vi "Voorbeeld_max_2_freq_detection.vi"() -> ()   [LabVIEW 2019]
uses:
  <vilib>/express/express analysis/Spectral/Block/exnSpectralBlock spectral measurements power poly.vi
  <vilib>/express/express analysis/Spectral/Block/exnSpectralBlock spectral measurements power DDT.vi
  <vilib>/express/express analysis/Spectral/XNode/ExpressSpectralMeasurementsBlockNode.xnode
panel:
  in  "Test Freq 2":dbl=1000.0 caption="Frequency"
  in  "Test Freq 1":dbl=500.0 caption="Frequency"
  in  "stop":bool
  out "Freq 2":i32
  out "Freq 1":i32
  out "Fourier Size":i32
  out "Waveform Graph 2":dynamicdata(graph)
  out "Frequency":dbl
  out "Waveform Graph":dynamicdata(graph)
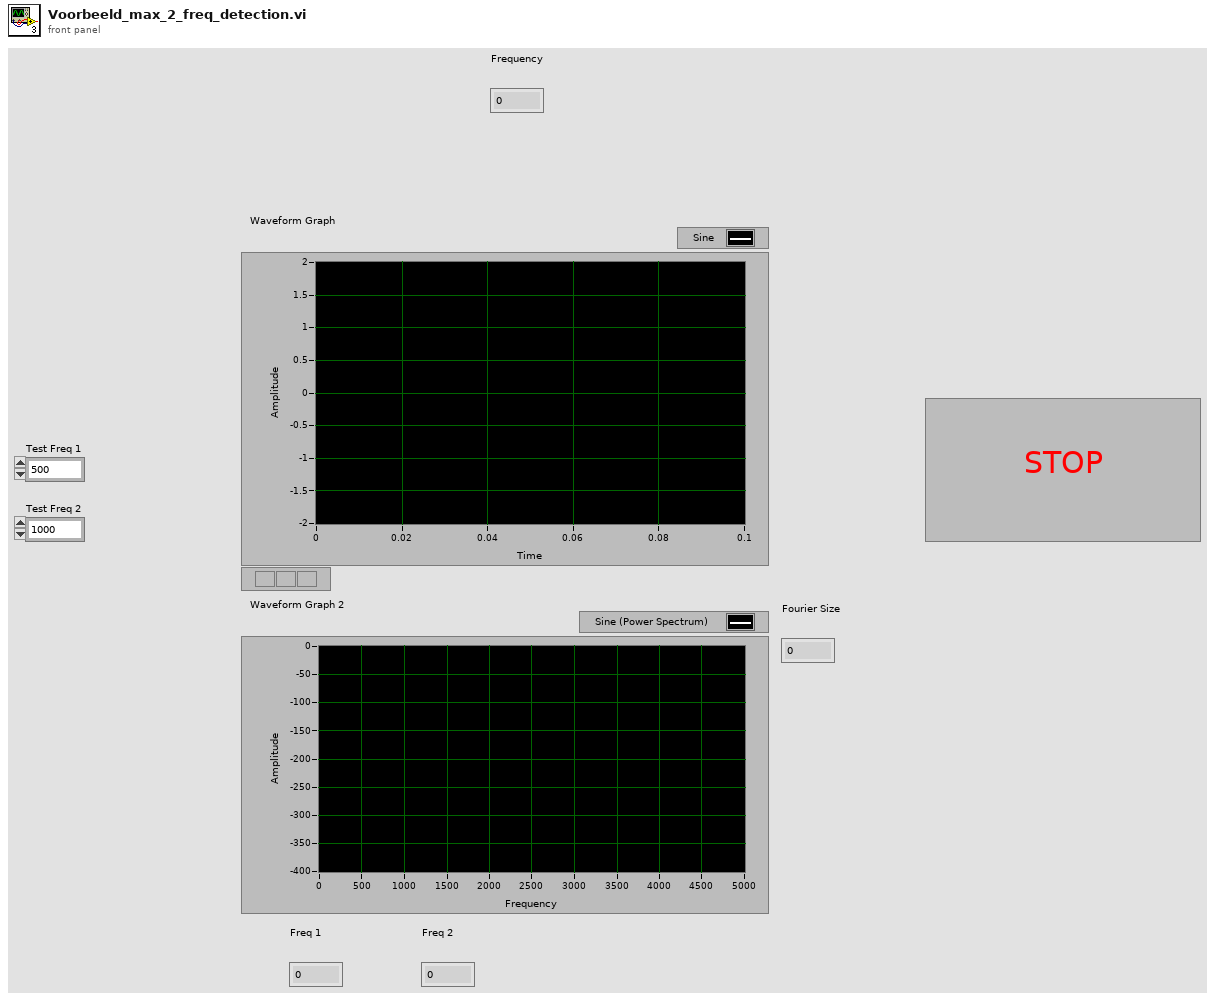
[diagram p1: front panel]
types:
  T1 = cluster{"averaging mode":u16, "weighting mode":u16, "number of averages":u32}
  T2 = cluster{"dB On (F)":bool, "unwrap phase (F)":bool, "convert to degree (F)":bool}
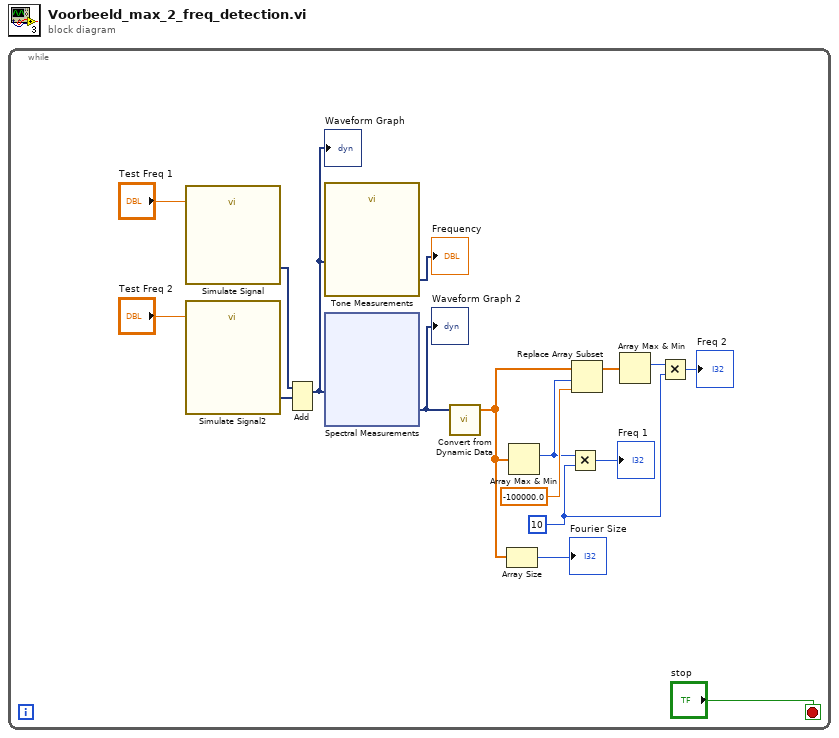
[diagram p0: block diagram]
diagram:
  n1 = while {
    stop <- "stop" stop-if-true
    w6 = 10 ("y")
    n2 = call "Simulate Signal"("Frequency"="Test Freq 1") -> ("Sine"=w17:dynamicdata)  [unwired: 13 in, 1 out]
    n3 = call "Simulate Signal2"("Frequency"="Test Freq 2") -> ("Sine"=w13:dynamicdata)  [unwired: 13 in, 1 out]
    n4 = Add(1:w13, 2:w17) -> (0:w14:dynamicdata)  [unwired: 1 in, 1 out]
    "Waveform Graph" <- w14
    n5 = call "Tone Measurements"("Signals"=w14) -> ("Frequency"=→"Frequency":dynamicdata)  [unwired: 9 in, 1 out]
    n6 = xnode "Spectral Measurements"("Signals"=w14) -> ("Power Spectrum"=w12:dynamicdata)  [unwired: 1 in, 1 out]
    "Waveform Graph 2" <- w12
    n7 = call "Convert from Dynamic Data"("Dynamic Data Type"=w12) -> ("Array"=w10:dbl[])  [unwired: 3 in]
    n8 = Array Size(array=w10) -> (size(s)=→"Fourier Size":i32)
    n9 = Array Max & Min(array=w10) -> (max index (indices)=w8:i32)  [unwired: 3 out]
    n10 = Multiply(x=w8, y=w6) -> (x*y=→"Freq 1":i32)
    n11 = Replace Array Subset(array=w10, new element=-100000.0 ("new element/subarray"), index=w8) -> (w9:dbl[])
    n12 = Array Max & Min(array=w9) -> (max index (indices)=w5:i32)  [unwired: 3 out]
    n13 = Multiply(x=w5, y=w6) -> (x*y=→"Freq 2":i32)
  }
